vi "RMET.vi"(2 "Run uninterrupted?":bool, 3 "Device Category IN:":string(combo)="Mini" caption="Device Category:", 5 "Sensor Serial No. IN:":string caption="Sensor Serial No.:", 6 "DB Serial No. IN:":string caption="DB Serial No.:") -> (0 "Done!":bool)   [LabVIEW 2019]
doc: "Performs IV measurements according to ATLAS ITk Quality Control Specifications."
uses:
  general_VIs/globals/QC_MeasurementSetup.vi
  general_VIs/globals/QC_RunInformation.vi
  InstrControl/InstrumentSetup.vi
  InstrControl/Switching/Switching.lvclass
  InstrControl/SupplyControl/SupplyControl.lvclass
  InstrControl/ArduinoControl/ArduinoControl.lvclass
  <vilib>/Analysis/NI_AALBase.lvlib
  InstrControl/InstrControl.lvclass
panel:
  out "Measurement Configuration Tab":enum32{"R_MET Setup", "R_MET Scan"}(tab)
  in  "Set voltage limit?":bool
  in  "Voltage Limit [mV]":dbl=1000.0 min=0.0001 format="%.3f"
  in  "Measurement Configurations":bool
  in  "Initial volts [uA] IN":dbl caption="Initial volts [V]"
  in  "Final volts [uA] IN":dbl=-700.0 caption="Final volts [V]"
  in  "step [uA] IN":dbl=10.0 caption="step [V]" format="%.1f"
  in  "step interval [s] IN":i32=10 caption="step interval [s]"
  in  "Continue":bool
  in  "Quit":bool
  out "RH":dbl[](array[numeric]) caption="RH [%]" format="%#.2f"
  out "Temp.":dbl[](array[numeric]) caption="Temp. [°C]" format="%#.2f"
  out "Resistance":dbl[](array[numeric]) caption="Resistance [Ohms]"
  out "Current":dbl[](array[numeric]) caption="Current [uA]"
  out "step interval [s]":i32=10
  out "step [V]":dbl=10.0 format="%.1f"
  out "Final volts [V]":dbl=-700.0 format="%.1f"
  out "Initial volts [V]":dbl format="%.1f"
  out "Igraph":cluster{dbl[], dbl[]}(graph)
  in  "Scales":T1(ring)
  in  "Iscale":enum16{"Ohms", "kiloOhms", "MegaOhms"}(ring)
  out "positive ramp?":bool
  out "DUT Description/Hardware Tab":enum32{"R_MET Setup", "R_MET Scan"}(tab)
  in  "Structure Name IN:":string caption="Structure Name:"
  in  "Switching":string(combo)="LXIPXI Switching"
  in  "Hardware Configurations":bool
  in  "User:":string(combo)="Xavi"
  in  "IV Supply":string(combo)="Keithley 2410"
  in  "Temperature":enum16{"Read Arduino", "Enter manually"}(ring)
  in  "Manufacturer:":string(combo)="Hamamatsu"
  out "Structure Name":string caption="Structure Name:"
  in  "abort":bool
  out "Device Category:":string
  out "DB Serial No.:":string
  out "Current Volts:":dbl format="%.2f"
  in  "quit (no save)":bool
  in  "Quit & Save":bool
  out "Bias On/Off:":bool
  out "STATUS 1":string
  out "Initiated:":string
  out "Sensor No.:":string
  out "No of steps":u32
  out "Current reading No.":u32
  out "Last reading at:":string
  # "University of\nCambridge"
  # "Strip Sensor QC: Metal Resistance"
  # "Vertical Scale:"
  # "Measurement Configuration"
  # "Scan parameters:"
  # "Last 5 readings:"
  # "n-4"
  # "n-3"
  # "n-2"
  # "n-1"
  # "n"
  # "DUT Description"
  # "Hardware"
  # "DUT & Test Description:"
  # "Current status:"
  # "Rdg No:"
  # "out of"
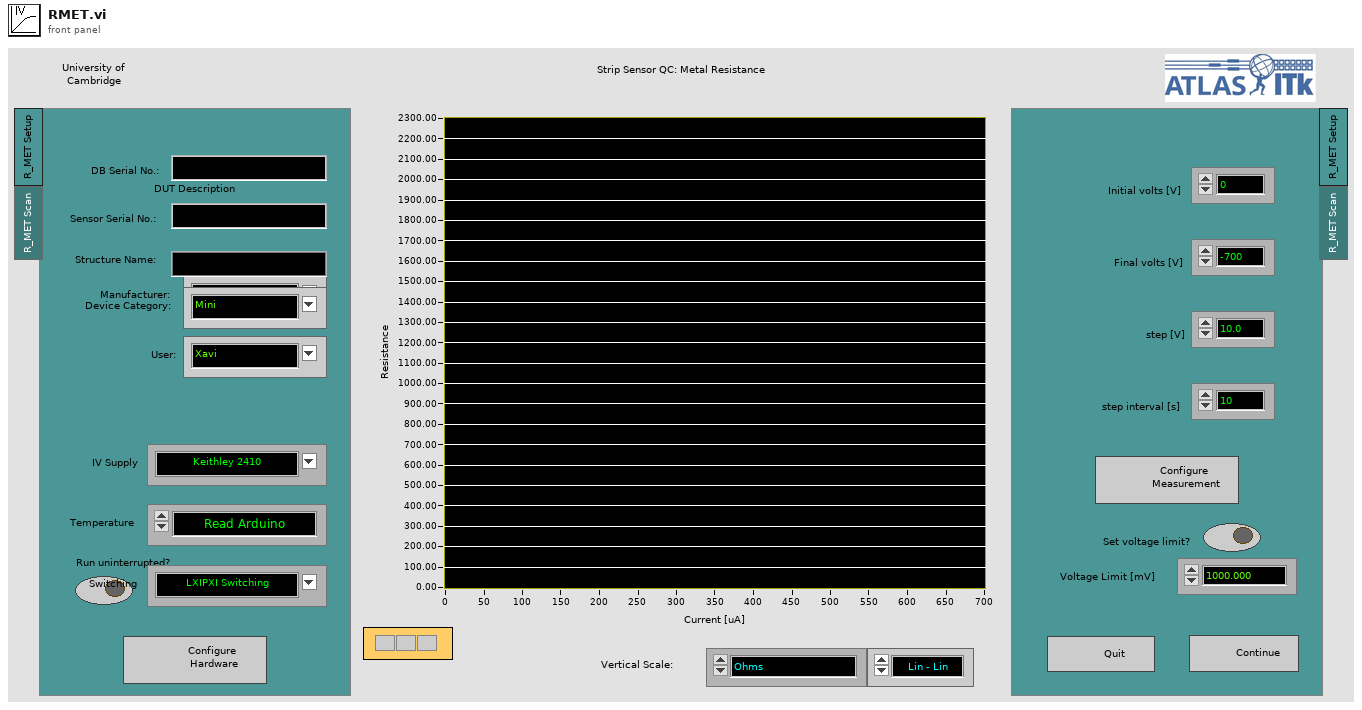
[diagram p1: front panel]
types:
  T1 = enum16{"Lin - Lin", "Log - Lin", "Lin - Log", "Log - log"}
  T2 = enum16{"Supply", "LCR", "Multimeter", "Switching"}
  T3 = enum16{"Reset", "Read Array", "Read Element", "Write Element", "Write Array", "Add Element", "Add Array"}
  T4 = enum16{"Reset", "Ground", "Striptest Bias", "Striptest SMU", "Striptest LCR", "IV", "CV", "Interstrip Cap", "Interstrip Res"}
  T5 = enum16{"Reset", "Ground", "Striptest Bias", "Striptest SMU", "Striptest LCR", "IV", "CV", "Interstrip Cap", "Interstrip Res", "PTP", "Implant Resistance", "Metal Resistance", "Coupling Capacitance"}
  T6 = cluster{"Supply":refnum<class "SupplyControl.lvclass">, "Initial Current [uA]":dbl, "Final Current [uA]":dbl, "Step Size [uA]":dbl, "Step Interval [s]":i32, "Number Of Steps":u32, "Ramp down steps [uA]":dbl, "Ramp down Interval [s]":i32, "Set Current Limit?":bool, "Voltage Limit [mV]":dbl, "Temperature Readout":enum16{"Read Arduino", "Enter manually"}, "Arduino":refnum<class "ArduinoControl.lvclass">, "Supply Name":string, "Switching":refnum<class "Switching.lvclass">, "Matrix used?":bool, "Matrix X Channels":cluster{"Bias Supply / SMU LO":i32, "Bias Supply / SMU HI":i32, "CV Box LO":i32, "CV Box HI":i32, "CV Box LO IN":i32, "CV Box HI IN":i32, "Volt meter LO":i32, "Volt meter HI":i32, "Mux1 C1":i32, "Mux1 C2":i32, "Mux2 C1":i32, "Mux2 C2":i32}, "Structure Name":string}
  T7 = cluster{"Sensor Serial No.:":string, "Wafer Serial No.:":string, "Batch:":string, "Manufacturer:":string, "Device Category:":string, "Database Serial No.:":string, "Date Initiated:":string, "Time Initiated:":string, "Test":string, "Instruments used:":string, "Probeplan used:":string, "End of Run comment:":string, "User:":string}
  T8 = cluster{"Institute":string, "Manufacturers":string[], "Devices":string[], "Serialnumbers Lookup DB":string, "Data directory":string, "Backup & screenshot directory":string, "List of known users":string[], "Measurement switch not used":bool, "Measurement Switch":string, "DUT Switch":string}
  T9 = cluster{"Supply":refnum<class "SupplyControl.lvclass">, "Initial Voltage [V]":dbl, "Final Voltage [V]":dbl, "Step Size [V]":dbl, "Step Interval [s]":i32, "Number Of Steps":u32, "Ramp down steps [V]":dbl, "Ramp down Interval [s]":i32, "Set Current Limit?":bool, "Current Limit [µA]":dbl, "Temperature Readout":enum16{"Read Arduino", "Enter manually"}, "Arduino":refnum<class "ArduinoControl.lvclass">, "Supply Name":string, "Switching":refnum<class "Switching.lvclass">, "Matrix used?":bool, "Matrix X Channels":cluster{"Bias Supply / SMU LO":i32, "Bias Supply / SMU HI":i32, "CV Box LO":i32, "CV Box HI":i32, "CV Box LO IN":i32, "CV Box HI IN":i32, "Volt meter LO":i32, "Volt meter HI":i32, "Mux1 C1":i32, "Mux1 C2":i32, "Mux2 C1":i32, "Mux2 C2":i32}, "Structure Name":string}
  T10 = cluster{"Voltage Limit":sgl, "R_Metal_KE2410":refnum<class "R_Metal_KE2410.lvclass">}
  T11 = cluster{"VISA address":refnum<visa-resource-name>, "T sensor":enum16{"SHT", "DS"}, "Arduino":refnum<class "ArduinoControl.lvclass">}
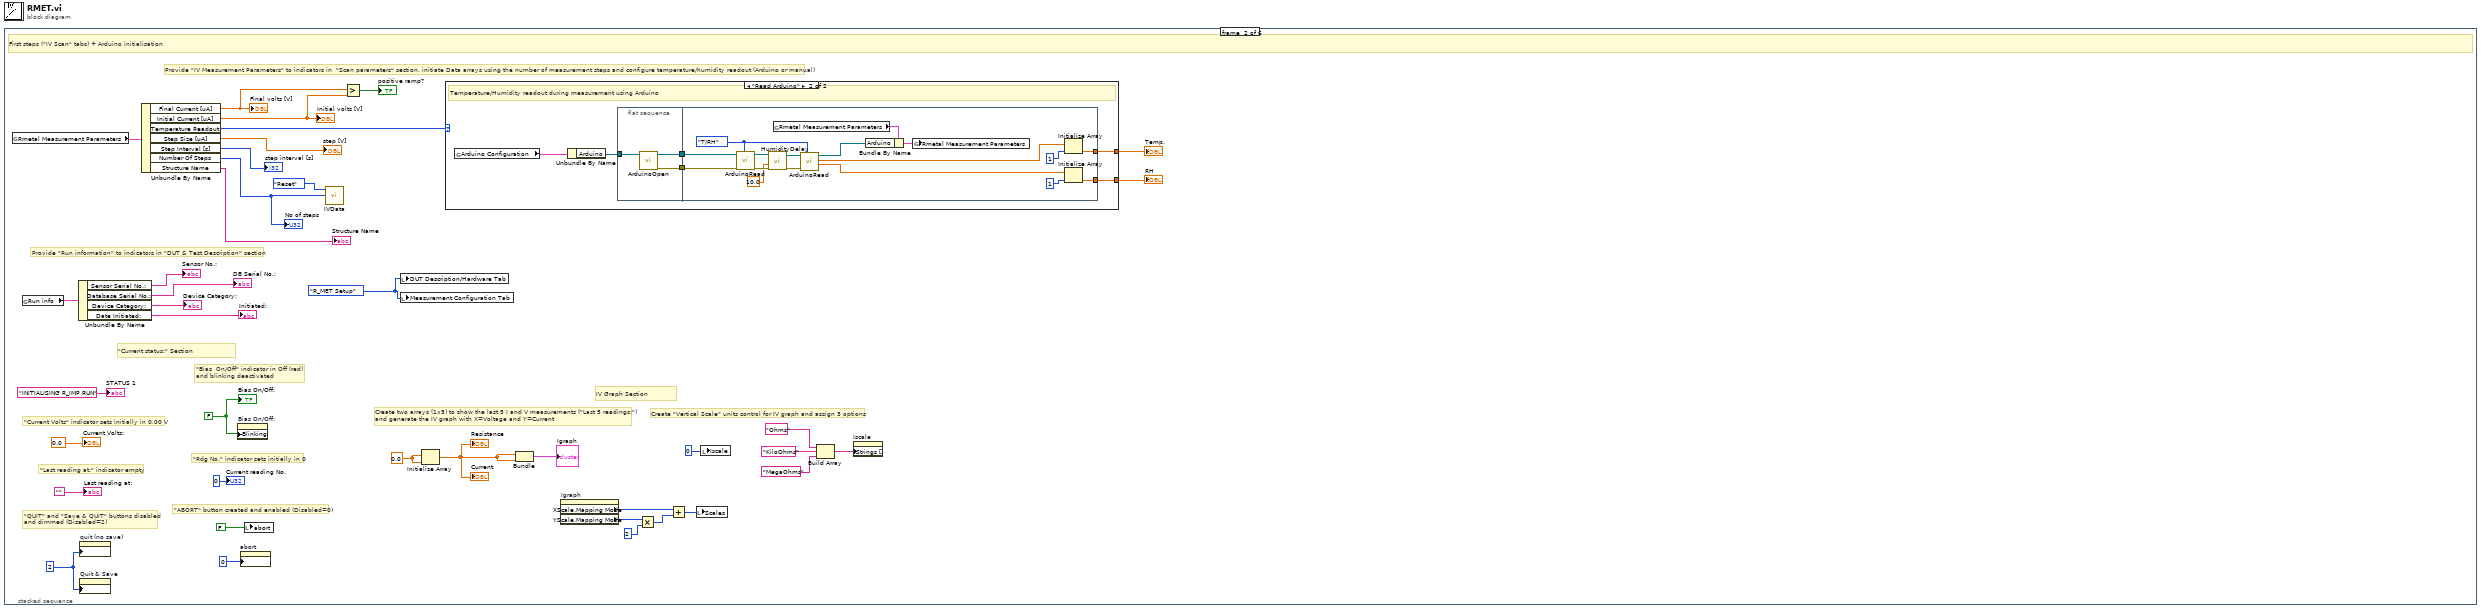
[diagram p0: block diagram]
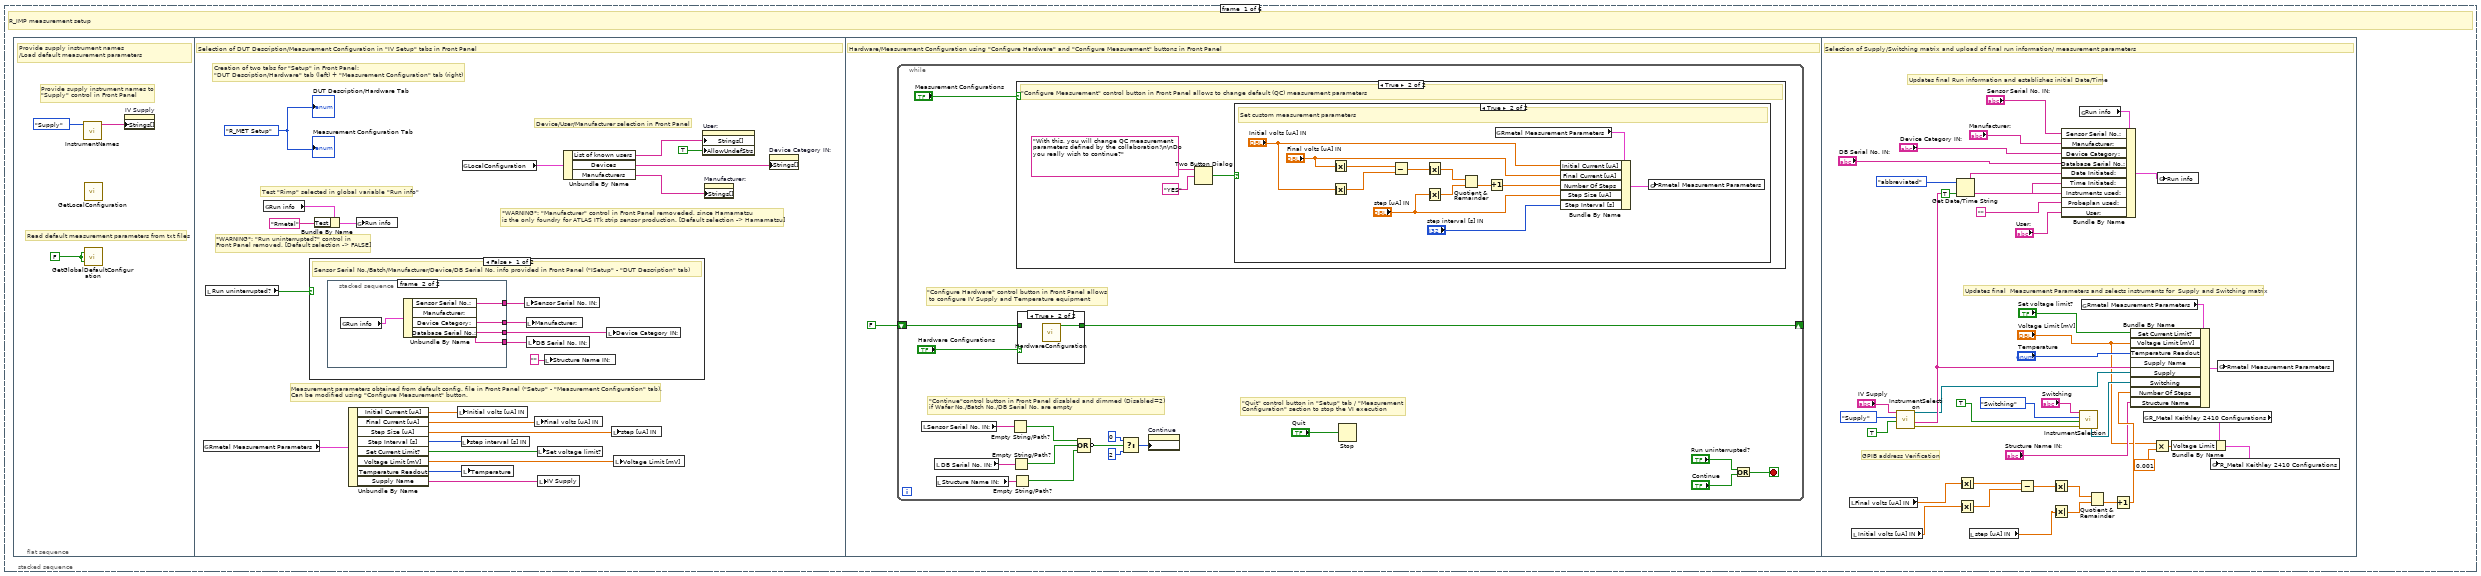
[diagram p2: hidden frame]
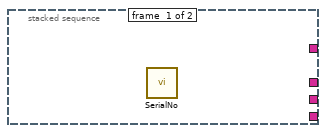
[diagram p3: hidden frame]
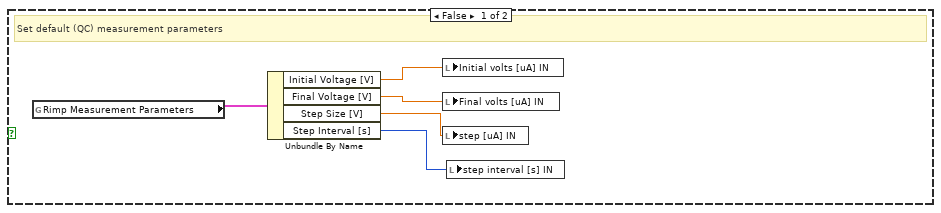
[diagram p6: hidden frame]
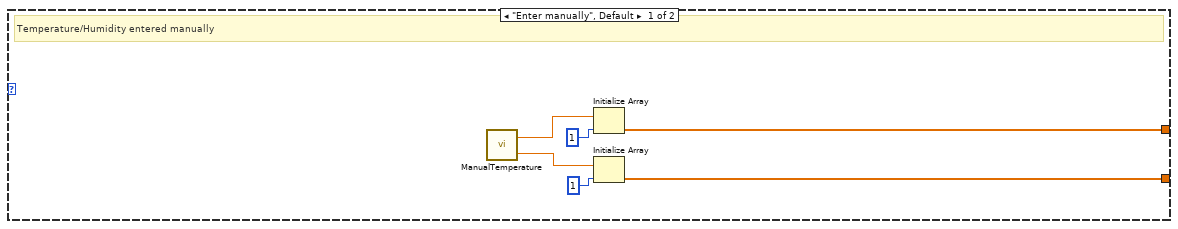
[diagram p8: hidden frame]
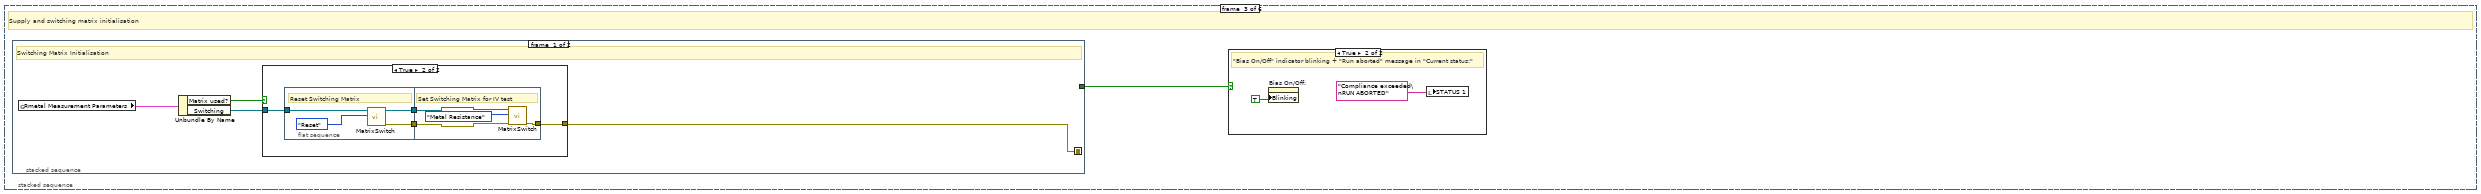
[diagram p9: hidden frame]
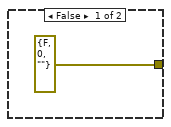
[diagram p10: hidden frame]
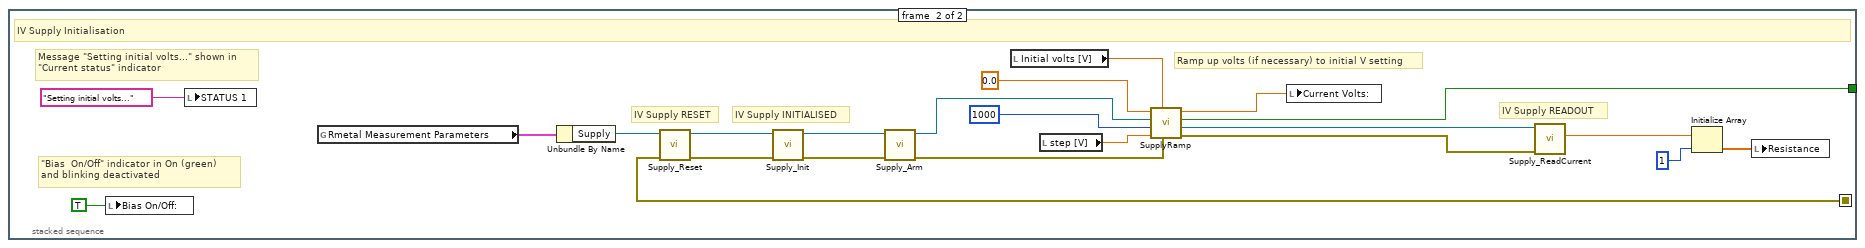
[diagram p11: hidden frame]
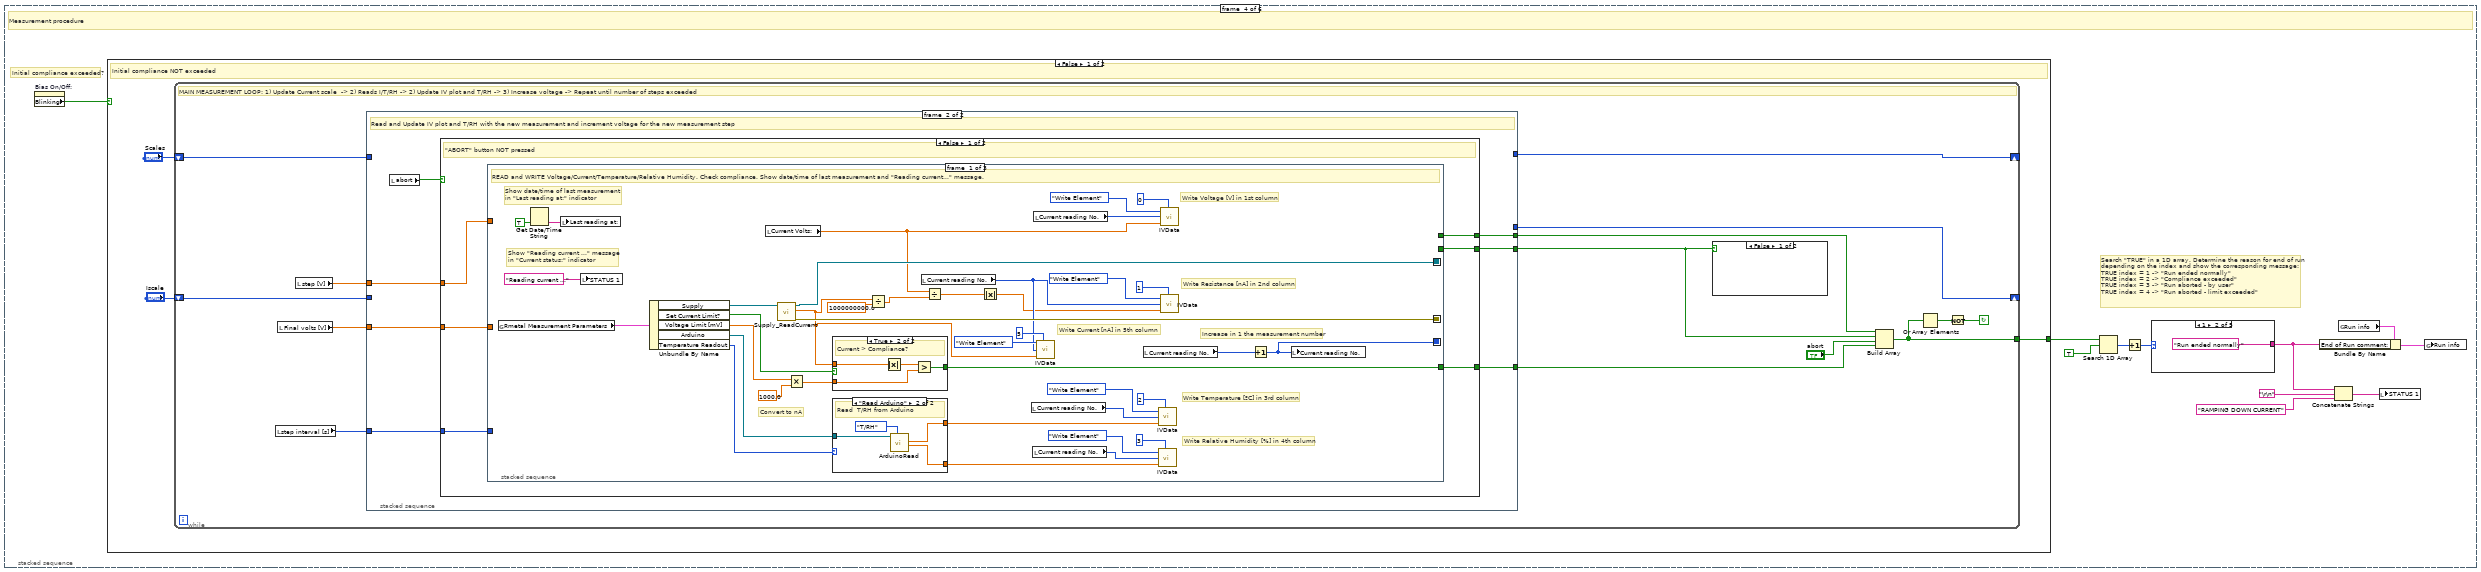
[diagram p13: hidden frame]
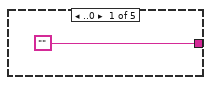
[diagram p14: hidden frame]
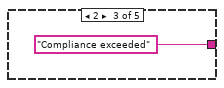
[diagram p15: hidden frame]
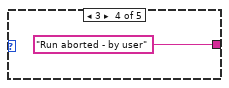
[diagram p16: hidden frame]
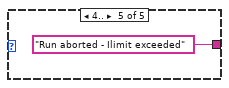
[diagram p17: hidden frame]
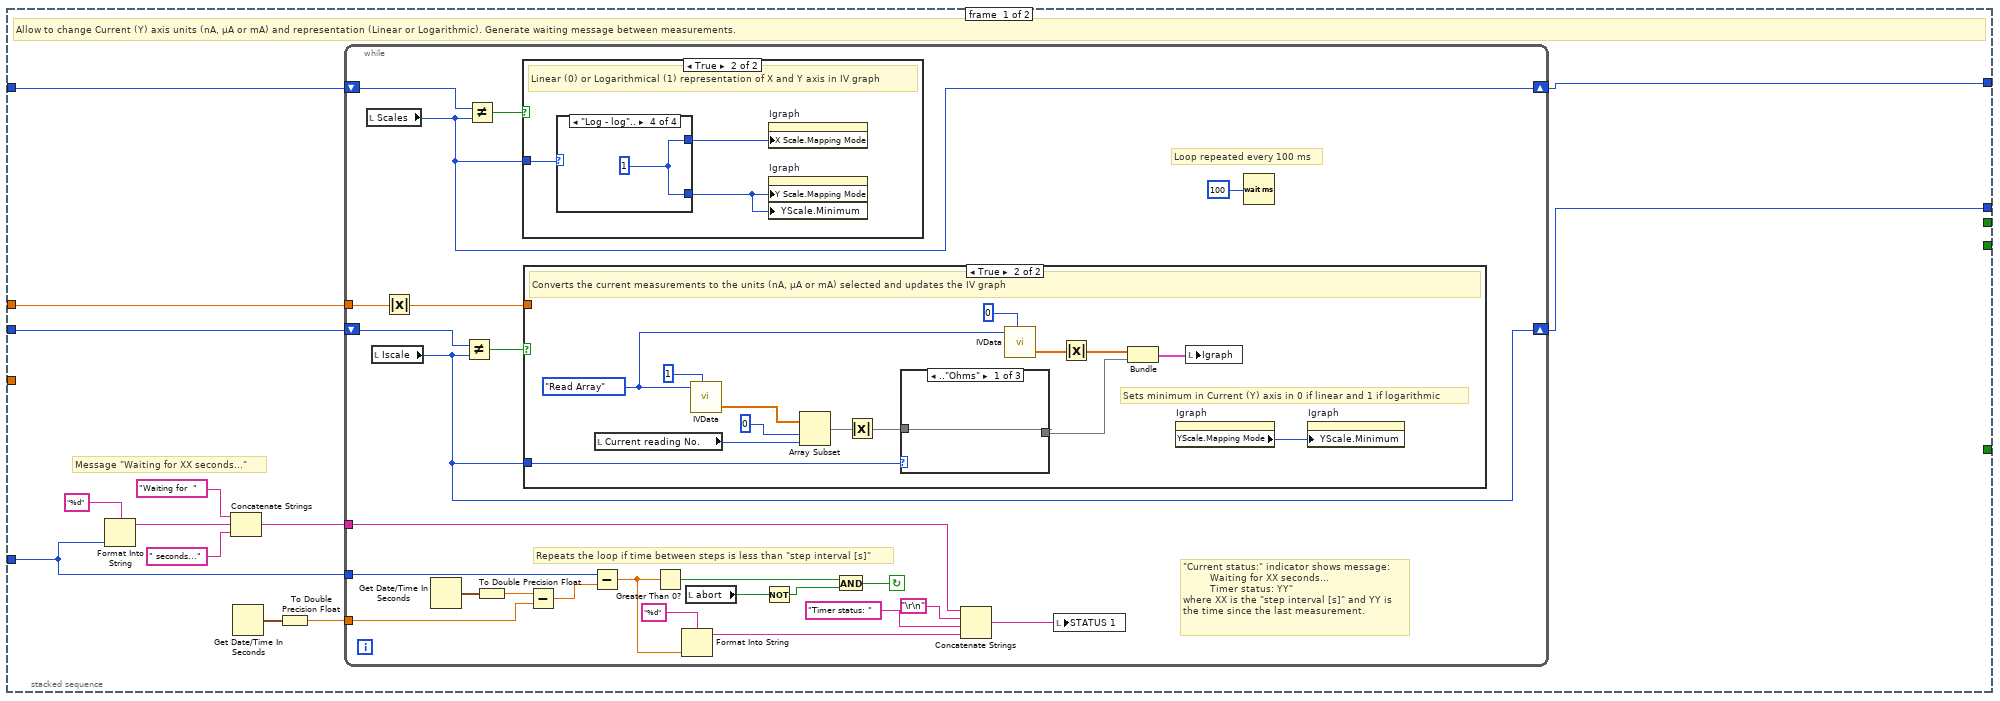
[diagram p18: hidden frame]
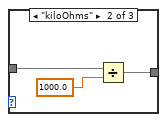
[diagram p20: hidden frame]
diagram:
  n1 = stacked-sequence {
    frame #0 {
      # "R_IMP measurement setup"
      n2 = flat-sequence {
        frame #0 {
          w3 = FALSE
          # "Read default measurement parameters from txt files"
          # "Provide supply instrument names to \n\"Supply\" control in Front Panel"
          # "Provide supply instrument names\n/Load default measurement parameters"
          n3 = call "InstrumentNames.vi"("Instrument type"=T2."Supply") -> ("Instrument names"=w1:string[])  [unwired: 9 in, 1 out]
          n4 = call "GetLocalConfiguration.vi"() -> ()  [unwired: 3 in, 1 out]
          n5 = call "GetGlobalDefaultConfiguration.vi"("DO NOT override instruments"=w3, "Read defaults?"=w3) -> ()  [unwired: 1 in, 1 out]
          n6 = property on="IV Supply" class="CmbBox"("Strings[]"=w1) -> ()  [unwired: 2 in, 2 out]
        }
        frame #1 {
          w4 = enum32{"R_MET Setup", "R_MET Scan"}."R_MET Setup" ("DUT Description/Hardware Tab")
          # "Device/User/Manufacturer selection in Front Panel"
          # "*WARNING*: \"Manufacturer\" control in Front Panel removeded, since Hamamatsu \nis the only foundry for ATLAS ITk strip sensor production. [Default selection -> Hamamatsu]"
          # "Measurement parameters obtained from default config. file in Front Panel (\"Setup\" - \"Measurement Configuration\" tab).\nCan be modified using \"Configure Measurement\" button."
          # "Test \"Rimp\" selected in global variable \"Run info\""
          # "Creation of two tabs for \"Setup\" in Front Panel:\n\"DUT Description/Hardware\" tab (left) + \"Measurement Configuration\" tab (right)"
          # "*WARNING*: \"Run uninterrupted?\" control in \nFront Panel removed. [Default selection -> FALSE]"
          # "Selection of DUT Description/Measurement Configuration in \"IV Setup\" tabs in Front Panel"
          n7 = global read "QC_MeasurementSetup.vi" "Rmetal Measurement Parameters"() -> (w20:T6)
          n8 = local read "Run uninterrupted?"() -> (w14:bool)
          n9 = global read "QC_RunInformation.vi" "Run info"() -> (w13:T7)
          n10 = case shown="False" w14 {
            frame False {
              # "Sensor Serial No./Batch/Manufacturer/Device/DB Serial No. info provided in Front Panel (\"ISetup\" - \"DUT Description\" tab)"
              n11 = stacked-sequence {
                tunnel: [_ w32] -> w26
                tunnel: [_ w31] -> w25
                tunnel: [_ w30] -> w27
                tunnel: [_ w28] -> w24
                frame #0 {
                  n12 = call "SerialNo.vi"() -> ()  [unwired: 5 in, 1 out]
                }
                frame #1 {
                  n13 = global read "QC_RunInformation.vi" "Run info"() -> (w29:T7)
                  n14 = Unbundle By Name(w29) -> ("Sensor Serial No.:"=w32:string, "Manufacturer:"=w31:string, "Device Category:"=w30:string, "Database Serial No.:"=w28:string)
                }
              }
              n15 = local write "Sensor Serial No. IN:"(w26) -> ()
              n16 = local write "Manufacturer:"(w25) -> ()
              n17 = local write "DB Serial No. IN:"(w24) -> ()
              n18 = local write "Structure Name IN:"("" ("Structure Name IN:")) -> ()
              n19 = local write "Device Category IN:"(w27) -> ()
            }
            frame True {
            }
          }
          n20 = Bundle By Name(cluster=w13, "Test"="Rmetal") -> (w12:T7)
          n21 = Unbundle By Name(w20) -> ("Initial Current [uA]"=w10:dbl, "Final Current [uA]"=w9:dbl, "Step Size [uA]"=w8:dbl, "Step Interval [s]"=w11:i32, "Set Current Limit?"=w19:bool, "Voltage Limit [mV]"=w18:dbl, "Temperature Readout"=w22:enum16{"Read Arduino", "Enter manually"}, "Supply Name"=w21:string)
          n22 = global write "QC_RunInformation.vi" "Run info"(w12) -> ()
          n23 = local write "Initial volts [uA] IN"(w10) -> ()
          n24 = local write "step interval [s] IN"(w11) -> ()
          n25 = local write "Temperature"(w22) -> ()
          n26 = global read "QC_RunInformation.vi" "LocalConfiguration"() -> (w17:T8)
          n27 = local write "Final volts [uA] IN"(w9) -> ()
          n28 = local write "Set voltage limit?"(w19) -> ()
          n29 = local write "IV Supply"(w21) -> ()
          n30 = Unbundle By Name(w17) -> ("List of known users"=w16:string[], "Devices"=w7:string[], "Manufacturers"=w6:string[])
          n31 = local write "step [uA] IN"(w8) -> ()
          n32 = local write "Voltage Limit [mV]"(w18) -> ()
          n33 = property on="User:" class="CmbBox"("Strings[]"=w16, "AllowUndefStrs"=TRUE) -> ()  [unwired: 2 in, 2 out]
          n34 = property on="Manufacturer:" class="CmbBox"("Strings[]"=w6) -> ()  [unwired: 2 in, 2 out]
          n35 = property on="Device Category IN:" class="CmbBox"("Strings[]"=w7) -> ()  [unwired: 2 in, 2 out]
          "DUT Description/Hardware Tab" <- w4
          "Measurement Configuration Tab" <- w4
        }
        frame #2 {
          # "Hardware/Measurement Configuration using \"Configure Hardware\" and \"Configure Measurement\" buttons in Front Panel"
          n36 = while {
            shift-right: [w43] -> _
            shift-left: FALSE -> [w42]
            stop <- w39 stop-if-true
            # "\"Continue\"control button in Front Panel disabled and dimmed (Disabled=2) \nif Wafer No./Batch No./DB Serial No. are empty"
            # "\"Configure Hardware\" control button in Front Panel allows\n to configure IV Supply and Temperature equipment"
            # "\"Quit\" control button in \"Setup\" tab / \"Measurement \nConfiguration\" section to stop the VI execution"
            n37 = local read "Sensor Serial No. IN:"() -> (w50:string)
            n38 = local read "DB Serial No. IN:"() -> (w37:string)
            n39 = local read "Structure Name IN:"() -> (w35:string)
            n40 = Empty String/Path?(string/path=w50) -> (empty?=w49:bool)
            n41 = Empty String/Path?(string/path=w37) -> (empty?=w36:bool)
            n42 = Empty String/Path?(string/path=w35) -> (empty?=w34:bool)
            n43 = case shown="True" "Measurement Configurations" {
              frame False {
              }
              frame True {
                # "\"Configure Measurement\" control button in Front Panel allows to change default (QC) measurement parameters"
                n44 = Two Button Dialog(message="With this, you will change QC measurement parameters defined by the collaboration!\n\nDo you really wish to continue?", 2:"YES") -> (T button?=w52:bool)  [unwired: 1 in]
                n45 = case shown="True" w52 {
                  frame False {
                    # "Set default (QC) measurement parameters"
                    n46 = global read "QC_MeasurementSetup.vi" "Rimp Measurement Parameters"() -> (w59:T9)
                    n47 = Unbundle By Name(w59) -> ("Initial Voltage [V]"=w57:dbl, "Final Voltage [V]"=w58:dbl, "Step Size [V]"=w56:dbl, "Step Interval [s]"=w55:i32)
                    n48 = local write "Initial volts [uA] IN"(w57) -> ()
                    n49 = local write "Final volts [uA] IN"(w58) -> ()
                    n50 = local write "step [uA] IN"(w56) -> ()
                    n51 = local write "step interval [s] IN"(w55) -> ()
                  }
                  frame True {
                    # "Set custom measurement parameters"
                    n52 = Absolute Value(x="Final volts [uA] IN") -> (abs(x)=w70:dbl)
                    n53 = Absolute Value(x="Initial volts [uA] IN") -> (abs(x)=w69:dbl)
                    n54 = Subtract(x=w70, y=w69) -> (x-y=w64:dbl)
                    n55 = Absolute Value(x=w64) -> (abs(x)=w66:dbl)
                    n56 = Absolute Value(x="step [uA] IN") -> (abs(x)=w65:dbl)
                    n57 = Quotient & Remainder(x=w66, y=w65) -> (floor(x/y)=w63:dbl)  [unwired: 1 out]
                    n58 = Increment(x=w63) -> (x+1=w62:dbl)
                    n59 = global read "QC_MeasurementSetup.vi" "Rmetal Measurement Parameters"() -> (w72:T6)
                    n60 = Bundle By Name(cluster=w72, "Initial Current [uA]"="Initial volts [uA] IN", "Final Current [uA]"="Final volts [uA] IN", "Number Of Steps"=w62, "Step Size [uA]"="step [uA] IN", "Step Interval [s]"="step interval [s] IN") -> (w71:T6)
                    n61 = global write "QC_MeasurementSetup.vi" "Rmetal Measurement Parameters"(w71) -> ()
                  }
                }
              }
            }
            n62 = case shown="True" "Hardware Configurations" {
              tunnel: [w73 w74] -> w43
              tunnel: w42 -> [w73 _]
              frame False {
              }
              frame True {
                n63 = call "HardwareConfiguration.vi"() -> ("configured?"=w74:bool)  [unwired: 11 in]
              }
            }
            n64 = Compound Arithmetic op=OR(w49, w36, w34) -> (invert w48:bool)
            n65 = Select(t=0, s=w48, f=2) -> (s? t:f=w45:i32)
            n66 = property on="Continue" class="Bool"("DisabledEnum"=w45) -> ()  [unwired: 2 in, 2 out]
            n67 = Stop(stop? (T)="Quit") -> ()
            n68 = Or(x="Run uninterrupted?", y="Continue") -> (x .or. y?=w39:bool)
          }
        }
        frame #3 {
          # "GPIB address Verification"
          # "Updates final  Measurement Parameters and selects instruments for  Supply and Switching matrix"
          # "Updates final Run information and establishes initial Date/Time"
          # "Selection of Supply/Switching matrix and upload of final run information/ measurement parameters"
          n69 = local read "Final volts [uA] IN"() -> (w82:dbl)
          n70 = local read "Initial volts [uA] IN"() -> (w83:dbl)
          n71 = call "InstrumentSelection.vi"("Verify GPIB address"=TRUE, "Instrument type"=T2."Supply", "Instrument name IN"="IV Supply") -> ("error out"=w100:errorcluster, "Instrument name OUT"=w103:string, "Supply"=w102:refnum<class "SupplyControl.lvclass">)  [unwired: 3 in, 3 out]
          n72 = Get Date/Time String(date format (0)=enum16{"short", "long", "abbreviated"}."abbreviated", want seconds? (F)=TRUE) -> (date string=w94:string, time string=w93:string)  [unwired: 1 in]
          n73 = Absolute Value(x=w82) -> (abs(x)=w90:dbl)
          n74 = Absolute Value(x=w83) -> (abs(x)=w89:dbl)
          n75 = local read "step [uA] IN"() -> (w84:dbl)
          n76 = Subtract(x=w90, y=w89) -> (x-y=w86:dbl)
          n77 = Absolute Value(x=w86) -> (abs(x)=w88:dbl)
          n78 = Absolute Value(x=w84) -> (abs(x)=w87:dbl)
          n79 = global read "QC_RunInformation.vi" "Run info"() -> (w111:T7)
          n80 = Bundle By Name(cluster=w111, "Sensor Serial No.:"="Sensor Serial No. IN:", "Manufacturer:"="Manufacturer:", "Device Category:"="Device Category IN:", "Database Serial No.:"="DB Serial No. IN:", "Date Initiated:"=w94, "Time Initiated:"=w93, "Instruments used:"=w103, "Probeplan used:"="", "User:"="User:") -> (w110:T7)
          n81 = call "InstrumentSelection.vi"("error in (no error)"=w100, "Verify GPIB address"=TRUE, "Instrument type"=T2."Switching", "Instrument name IN"="Switching") -> ("Switching"=w99:refnum<class "Switching.lvclass">)  [unwired: 2 in, 5 out]
          n82 = global read "QC_MeasurementSetup.vi" "Rmetal Measurement Parameters"() -> (w115:T6)
          n83 = Quotient & Remainder(x=w88, y=w87) -> (floor(x/y)=w85:dbl)  [unwired: 1 out]
          n84 = Increment(x=w85) -> (x+1=w81:dbl)
          n85 = Bundle By Name(cluster=w115, "Set Current Limit?"="Set voltage limit?", "Voltage Limit [mV]"="Voltage Limit [mV]", "Temperature Readout"="Temperature", "Supply Name"=w103, "Supply"=w102, "Switching"=w99, "Number Of Steps"=w81, "Structure Name"="Structure Name IN:") -> (w116:T6)
          n86 = global read "InstrumentSetup.vi" "R_Metal Keithley 2410 Configurations"() -> (w79:T10)
          n87 = Multiply(x="Voltage Limit [mV]", y=0.001) -> (x*y=w76:dbl)
          n88 = global write "QC_RunInformation.vi" "Run info"(w110) -> ()
          n89 = Bundle By Name(cluster=w79, "Voltage Limit"=w76) -> (w78:T10)
          n90 = global write "InstrumentSetup.vi" "R_Metal Keithley 2410 Configurations"(w78) -> ()
          n91 = global write "QC_MeasurementSetup.vi" "Rmetal Measurement Parameters"(w116) -> ()
        }
      }
    }
    frame #1 {
      w117 = enum32{"R_MET Setup", "R_MET Scan"}."R_MET Setup" ("DUT Description/Hardware Tab")
      w139 = 2
      w145 = 0.0
      w138 = FALSE ("Visible")
      # "IV Graph Section"
      # "\"Current status:\" Section"
      # "Create two arrays (1x5) to show the last 5 I and V measurements (\"Last 5 readings:\") \nand generate the IV graph with X=Voltage and Y=Current"
      # "\"Bias  On/Off\" indicator in Off (red)\nand blinking deactivated"
      # "\"Rdg No.\" indicator sets initially in 0"
      # "\"ABORT\" button created and enabled (Disabled=0)"
      # "\"Current Volts\" indicator sets initially in 0.00 V"
      # "\"Last reading at:\" indicator empty"
      # "\"QUIT\" and \"Save & QUIT\" buttons disabled\nand dimmed (Disabled=2)"
      # "Create \"Vertical Scale\" units control for IV graph and assign 3 options"
      # "Provide \"Run information\" to indicators in \"DUT & Test Description\" section"
      # "Provide \"IV Measurement Parameters\" to indicators in  \"Scan parameters\" section, initiate Data arrays using the number of measurement steps and configure temperature/humidity readout (Arduino or manual)"
      # "First steps (\"IV Scan\" tabs) + Arduino initialisation"
      n92 = global read "QC_MeasurementSetup.vi" "Rmetal Measurement Parameters"() -> (w129:T6)
      n93 = global read "QC_RunInformation.vi" "Run info"() -> (w154:T7)
      n94 = Unbundle By Name(w154) -> ("Sensor Serial No.:"=→"Sensor No.:":string, "Database Serial No.:"=→"DB Serial No.:":string, "Device Category:"=→"Device Category:":string, "Date Initiated:"=→"Initiated:":string)
      n95 = property on="quit (no save)" class="Bool"("DisabledEnum"=w139) -> ()  [unwired: 2 in, 2 out]
      n96 = property on="Quit & Save" class="Bool"("DisabledEnum"=w139) -> ()  [unwired: 2 in, 2 out]
      n97 = Unbundle By Name(w129) -> ("Final Current [uA]"=w121:dbl, "Initial Current [uA]"=w122:dbl, "Temperature Readout"=w123:enum16{"Read Arduino", "Enter manually"}, "Step Size [uA]"=→"step [V]":dbl, "Step Interval [s]"=→"step interval [s]":i32, "Number Of Steps"=w119:u32, "Structure Name"=→"Structure Name":string)
      "No of steps" <- w119
      "Initial volts [V]" <- w122
      "Final volts [V]" <- w121
      n98 = property on="Bias On/Off:" class="Bool (strict)"("Blinking"=w138) -> ()  [unwired: 2 in, 2 out]
      n99 = property on="abort" class="Bool (strict)"("DisabledEnum"=0) -> ()  [unwired: 2 in, 2 out]
      n100 = local write "abort"(FALSE) -> ()
      n101 = call "IVData.vi"("Action"=T3."Reset", "Array Size / Index"=w119) -> ()  [unwired: 3 in, 2 out]
      n102 = Greater?(x=w121, y=w122) -> (0:→"positive ramp?":bool)
      n103 = local write "DUT Description/Hardware Tab"(w117) -> ()
      n104 = local write "Measurement Configuration Tab"(w117) -> ()
      n105 = Initialize Array(w145, w145) -> (w125:dbl[])
      "Current" <- w125
      "Resistance" <- w125
      n106 = case shown="\"Read Arduino\"" w123 {
        tunnel: [w160 w167] -> w142
        tunnel: [w157 w166] -> w130
        frame "Enter manually", Default {
          # "Temperature/Humidity entered manually"
          n107 = call "ManualTemperature.vi"() -> ("Humidity [%] out"=w156:dbl, "Temperature [°C] out"=w161:dbl)
          n108 = Initialize Array(w161, 1) -> (w160:dbl[])
          n109 = Initialize Array(w156, 1) -> (w157:dbl[])
        }
        frame "Read Arduino" {
          # "Temperature/Humidity readout during measurement using Arduino"
          n110 = global read "InstrumentSetup.vi" "Arduino Configuration"() -> (w163:T11)
          n111 = Unbundle By Name(w163) -> ("Arduino"=w162:refnum<class "ArduinoControl.lvclass">)
          n112 = flat-sequence {
            tunnel: [w168] -> w165
            tunnel: [w170] -> w164
            tunnel: w162 -> [w169]
            tunnel: [w187] -> w167
            tunnel: [w184] -> w166
            tunnel: w165 -> [w178]
            tunnel: w164 -> [w177]
            frame #0 {
              n113 = call "ArduinoOpen.vi"("ArduinoControl in"=w169) -> ("error out"=w170:errorcluster, "ArduinoControl out"=w168:refnum<class "ArduinoControl.lvclass">)  [unwired: 9 in]
            }
            frame #1 {
              w176 = enum16{"T/RH", "Interlock", "Edgesense"}."T/RH" ("Arduino function")
              n114 = call "ArduinoRead.vi"("Arduino function"=w176, "error in (no error)"=w177, "ArduinoControl in"=w178) -> ("error out"=w172:errorcluster, "ArduinoControl out"=w173:refnum<class "ArduinoControl.lvclass">)  [unwired: 3 in, 4 out]
              n115 = call "HumidityDelay.vi"("error in (no error)"=w172, "Start Humidity"=10.0, "ArduinoControl in"=w173) -> ("error out"=w175:errorcluster, "ArduinoControl out"=w174:refnum<class "ArduinoControl.lvclass">)  [unwired: 7 in]
              n116 = global read "QC_MeasurementSetup.vi" "Rmetal Measurement Parameters"() -> (w180:T6)
              n117 = call "ArduinoRead.vi"("Arduino function"=w176, "error in (no error)"=w175, "ArduinoControl in"=w174) -> ("rel. Humidity [%]"=w182:dbl, "Temperature [°C]"=w183:dbl, "ArduinoControl out"=w181:refnum<class "ArduinoControl.lvclass">)  [unwired: 3 in, 3 out]
              n118 = Bundle By Name(cluster=w180, "Arduino"=w181) -> (w179:T6)
              n119 = global write "QC_MeasurementSetup.vi" "Rmetal Measurement Parameters"(w179) -> ()
              n120 = Initialize Array(w183, 1) -> (w187:dbl[])
              n121 = Initialize Array(w182, 1) -> (w184:dbl[])
            }
          }
        }
      }
      "Temp." <- w142
      "RH" <- w130
      n122 = Bundle(w125, w125) -> (→"Igraph":cluster{dbl[], dbl[]})  [unwired: 1 in]
      n123 = property on="Igraph" class="XYGraph (strict)"() -> ("XScale.Mapping Mode"=w133:u8, "YScale.Mapping Mode"=w132:u8)  [unwired: 2 in, 2 out]
      n124 = Multiply(x=w132, y=2) -> (x*y=w135:i32)
      n125 = Add(x=w133, y=w135) -> (x+y=w131:i32)
      n126 = local write "Scales"(w131) -> ()
      n127 = local write "Iscale"(u16 0 ("Scale")) -> ()
      n128 = Build Array("Ohms", "KiloOhms", "MegaOhms") -> (w151:string[])
      n129 = property on="Iscale" class="Enum (strict)"("Strings []"=w151) -> ()  [unwired: 2 in, 2 out]
      "STATUS 1" <- "INITIALISING R_IMP RUN"
      "Bias On/Off:" <- w138
      "Last reading at:" <- ""
      "Current reading No." <- u32 0 ("Current reading No.")
      "Current Volts:" <- 0.0 ("Current Volts:")
    }
    frame #2 {
      # "Supply and switching matrix initialisation"
      n130 = stacked-sequence {
        seq-local: [w190 _] -> [_ w206]
        tunnel: [_ w207] -> w188
        frame #0 {
          # "Switching Matrix Initialisation"
          n131 = global read "QC_MeasurementSetup.vi" "Rmetal Measurement Parameters"() -> (w189:T6)
          n132 = Unbundle By Name(w189) -> ("Matrix used?"=w192:bool, "Switching"=w191:refnum<class "Switching.lvclass">)
          n133 = case shown="True" w192 {
            tunnel: w191 -> [_ w194]
            tunnel: [errorcluster {"status"=FALSE, "code"=0, "source"=""} ("error constant") w195] -> w190
            frame False {
            }
            frame True {
              n134 = flat-sequence {
                tunnel: [w201] -> w197
                tunnel: [w200] -> w196
                tunnel: w194 -> [w199]
                tunnel: w197 -> [w205]
                tunnel: w196 -> [w204]
                tunnel: [w203] -> w195
                frame #0 {
                  # "Reset Switching Matrix"
                  n135 = call-dynamic "MatrixSwitch.vi"("Action"=T4."Reset", "Switching in"=w199) -> ("error out"=w201:errorcluster, "Switching out"=w200:refnum<class "Switching.lvclass">)  [unwired: 7 in, 1 out]
                }
                frame #1 {
                  # "Set Switching Matrix for IV test"
                  n136 = call-dynamic "MatrixSwitch.vi"("error in (no error)"=w205, "Action"=T5."Metal Resistance", "Switching in"=w204) -> ("error out"=w203:errorcluster)  [unwired: 6 in, 2 out]
                }
              }
            }
          }
        }
        frame #1 {
          # "IV Supply READOUT"
          # "IV Supply INITIALISED"
          # "IV Supply RESET"
          # "Message \"Setting initial volts...\" shown in \n\"Current status\" indicator"
          # "\"Bias  On/Off\" indicator in On (green)\nand blinking deactivated"
          # "Ramp up volts (if necessary) to initial V setting"
          # "IV Supply Initialisation"
          n137 = local write "Bias On/Off:"(TRUE ("Compliance?")) -> ()
          n138 = local write "STATUS 1"("Setting initial volts..." ("STATUS 1")) -> ()
          n139 = global read "QC_MeasurementSetup.vi" "Rmetal Measurement Parameters"() -> (w223:T6)
          n140 = Unbundle By Name(w223) -> ("Supply"=w220:refnum<class "SupplyControl.lvclass">)
          n141 = call-dynamic "Supply_Reset.vi"("error in (no error)"=w206, "SupplyControl in"=w220) -> ("error out"=w225:errorcluster, "SupplyControl out"=w227:refnum<class "SupplyControl.lvclass">)  [unwired: 8 in]
          n142 = call-dynamic "Supply_Init.vi"("error in (no error)"=w225, "SupplyControl in"=w227) -> ("error out"=w224:errorcluster, "SupplyControl out"=w226:refnum<class "SupplyControl.lvclass">)  [unwired: 8 in]
          n143 = call-dynamic "Supply_Arm.vi"("error in (no error)"=w224, "SupplyControl in"=w226) -> ("error out"=w213:errorcluster, "SupplyControl out"=w214:refnum<class "SupplyControl.lvclass">)  [unwired: 8 in]
          n144 = local read "Initial volts [V]"() -> (w215:dbl)
          n145 = local read "step [V]"() -> (w216:dbl)
          n146 = call "SupplyRamp.vi"("error in"=w213, "Requested Voltage"=w215, "Step Size"=w216, "Step Delay"=1000, "Supply IN"=w214, "Starting Voltage"=0.0) -> ("error out"=w208:errorcluster, "Supply OUT"=w209:refnum<class "SupplyControl.lvclass">, "Compliance exceeded"=w207:bool, "Current Voltage"=w219:dbl)  [unwired: 2 in]
          n147 = local write "Current Volts:"(w219) -> ()
          n148 = call-dynamic "Supply_ReadCurrent.vi"("error in (no error)"=w208, "SupplyControl in"=w209) -> ("Current in nA"=w211:dbl)  [unwired: 7 in, 2 out]
          n149 = Initialize Array(w211, 1) -> (w210:dbl[])
          n150 = local write "Resistance"(w210) -> ()
        }
      }
      n151 = case shown="True" w188 {
        frame False {
        }
        frame True {
          # "\"Bias On/Off\" indicator blinking + \"Run aborted\" message in \"Current status:\""
          n152 = property on="Bias On/Off:" class="Bool (strict)"("Blinking"=TRUE) -> ()  [unwired: 2 in, 2 out]
          n153 = local write "STATUS 1"("Compliance exceeded\nRUN ABORTED") -> ()
        }
      }
    }
    frame #3 {
      # "Search \"TRUE\" in a 1D array. Determine the reason for end of run \ndepending on the index and show the corresponding message:\nTRUE index = 1 -> \"Run ended normally\"\nTRUE index = 2 -> \"Compliance exceeded\"\nTRUE index = 3 -> \"Run aborted - by user\"\nTRUE index = 4 -> \"Run aborted - limit exceeded\""
      # "Initial compliance exceeded?"
      # "Measurement procedure"
      n154 = property on="Bias On/Off:" class="Bool (strict)"() -> ("Blinking"=w240:bool)  [unwired: 2 in, 2 out]
      n155 = case shown="False" w240 {
        tunnel: [w248 w494] -> w239
        frame False {
          # "Initial compliance NOT exceeded"
          n156 = while {
            shift-left: "Iscale" -> [w258]
            shift-right: [w257] -> _
            shift-left: "Scales" -> [w259]
            shift-right: [w260] -> _
            tunnel: [w256] -> w248
            stop <- w261 continue-if-true
            # "MAIN MEASUREMENT LOOP: 1) Update Current scale  -> 2) Reads I/T/RH -> 2) Update IV plot and T/RH -> 3) Increase voltage -> Repeat until number of steps exceeded"
            n157 = local read "step interval [s]"() -> (w253:i32)
            n158 = local read "Final volts [V]"() -> (w254:dbl)
            n159 = local read "step [V]"() -> (w255:dbl)
            n160 = stacked-sequence {
              tunnel: [w275 _] -> w260
              tunnel: w255 -> [w272 w337]
              tunnel: [_ w336] -> w251
              tunnel: w254 -> [_ w335]
              tunnel: w253 -> [w263 w334]
              tunnel: [_ w333] -> w252
              tunnel: w259 -> [w274 _]
              tunnel: w258 -> [w273 _]
              tunnel: [w271 _] -> w257
              tunnel: [_ w331] -> w249
              frame #0 {
                # "Message \"Waiting for XX seconds...\""
                # "Allow to change Current (Y) axis units (nA, µA or mA) and representation (Linear or Logarithmic). Generate waiting message between measurements."
                n161 = Format Into String(format string="%d", w263) -> (resulting string=w268:string)  [unwired: 2 in, 1 out]
                n162 = Concatenate Strings("Waiting for  ", w268, " seconds...") -> (w264:string)
                n163 = Get Date/Time In Seconds() -> (seconds since 1Jan1904=w265:timestamp)
                n164 = To Double Precision Float(number=w265) -> (double precision float=w266:dbl)
                n165 = while {
                  tunnel: w272 -> [w284]
                  shift-left: w273 -> [w288]
                  shift-right: [w281] -> w271
                  shift-left: w274 -> [w289]
                  shift-right: [w290] -> w275
                  tunnel: w264 -> [w282]
                  tunnel: w263 -> [w294]
                  tunnel: w266 -> [w295]
                  stop <- w296 continue-if-true
                  # "\"Current status:\" indicator shows message:\n         Waiting for XX seconds...\n         Timer status: YY\"\nwhere XX is the \"step interval [s]\" and YY is\nthe time since the last measurement."
                  # "Repeats the loop if time between steps is less than \"step interval [s]\""
                  # "Loop repeated every 100 ms"
                  n166 = local read "Scales"() -> (w290:T1)
                  n167 = local read "Iscale"() -> (w281:enum16{"Ohms", "kiloOhms", "MegaOhms"})
                  n168 = Absolute Value(x=w284) -> (abs(x)=w283:dbl)
                  n169 = Get Date/Time In Seconds() -> (seconds since 1Jan1904=w280:timestamp)
                  n170 = Not Equal?(x=w288, y=w281) -> (x != y?=w279:bool)
                  n171 = Not Equal?(x=w289, y=w290) -> (x != y?=w291:bool)
                  n172 = To Double Precision Float(number=w280) -> (double precision float=w300:dbl)
                  n173 = case shown="True" w291 {
                    tunnel: w290 -> [_ w324]
                    frame False {
                    }
                    frame True {
                      # "Linear (0) or Logarithmical (1) representation of X and Y axis in IV graph"
                      n174 = case shown="\"Log - log\".." w324 {
                        tunnel: [w325 1 0 w330] -> w323
                        tunnel: [w325 0 1 w330] -> w322
                        frame .."Lin - Lin" {
                          w325 = 0
                        }
                        frame "Log - Lin" {
                        }
                        frame "Lin - Log" {
                        }
                        frame "Log - log".. {
                          w330 = 1
                        }
                      }
                      n175 = property on="Igraph" class="XYGraph (strict)"("X Scale.Mapping Mode"=w323) -> ()  [unwired: 2 in, 2 out]
                      n176 = property on="Igraph" class="XYGraph (strict)"("Y Scale.Mapping Mode"=w322, "YScale.Minimum"=w322) -> ()  [unwired: 2 in, 2 out]
                    }
                  }
                  n177 = case shown="True" w279 {
                    tunnel: w283 -> [_ _]
                    tunnel: w281 -> [_ w309]
                    frame False {
                    }
                    frame True {
                      w303 = T3."Read Array" ("Action")
                      # "Sets minimum in Current (Y) axis in 0 if linear and 1 if logarithmic"
                      # "Converts the current measurements to the units (nA, µA or mA) selected and updates the IV graph"
                      n178 = local read "Current reading No."() -> (w311:u32)
                      n179 = call "IVData.vi"("Action"=w303, "Array No."=u32 1 ("Action")) -> ("Array OUT"=w312:dbl[])  [unwired: 3 in, 1 out]
                      n180 = Array Subset(array=w312, index=0, length=w311) -> (w308:dbl[])
                      n181 = Absolute Value(x=w308) -> (abs(x)=w307:dbl[])
                      n182 = case shown="..\"Ohms\"" w309 {
                        tunnel: [w315 w316 w320] -> w314
                        tunnel: w307 -> [w315 w318 w321]
                        frame .."Ohms" {
                        }
                        frame "kiloOhms" {
                          n183 = Divide(x=w318, y=1000.0) -> (x/y=w316:dbl[])
                        }
                        frame "MegaOhms".. {
                          n184 = Divide(x=w321, y=1000000.0) -> (x/y=w320:dbl[])
                        }
                      }
                      n185 = call "IVData.vi"("Action"=w303, "Array No."=u32 0 ("Action")) -> ("Array OUT"=w302:dbl[])  [unwired: 3 in, 1 out]
                      n186 = Absolute Value(x=w302) -> (abs(x)=w301:dbl[])
                      n187 = Bundle(w301, w314) -> (w310:cluster{dbl[], dbl[]})  [unwired: 1 in]
                      n188 = property on="Igraph" class="XYGraph (strict)"() -> ("YScale.Mapping Mode"=w305:u8)  [unwired: 2 in, 2 out]
                      n189 = local write "Igraph"(w310) -> ()
                      n190 = property on="Igraph" class="XYGraph (strict)"("YScale.Minimum"=w305) -> ()  [unwired: 2 in, 2 out]
                    }
                  }
                  n191 = Subtract(x=w300, y=w295) -> (x-y=w277:dbl)
                  n192 = Subtract(x=w294, y=w277) -> (x-y=w276:dbl)
                  n193 = Greater Than 0?(x=w276) -> (x > 0?=w278:bool)
                  n194 = Format Into String(format string="%d", w276) -> (resulting string=w298:string)  [unwired: 2 in, 1 out]
                  n195 = local read "abort"() -> (w293:bool)
                  n196 = Not(x=w293) -> (.not. x?=w299:bool)
                  n197 = And(x=w278, y=w299) -> (x .and. y?=w296:bool)
                  n198 = Concatenate Strings(w282, "\r\n", "Timer status: ", w298) -> (w292:string)
                  n199 = local write "STATUS 1"(w292) -> ()
                  n200 = Wait (ms)(milliseconds to wait=u32 100) -> ()  [unwired: 1 out]
                }
              }
              frame #1 {
                # "Read and Update IV plot and T/RH with the new measurement and increment voltage for the new measurement step"
                n201 = local read "abort"() -> (w332:bool)
                n202 = case shown="False" w332 {
                  tunnel: [w343 w491] -> w333
                  tunnel: w334 -> [w342 _]
                  tunnel: w335 -> [w341 _]
                  tunnel: [w339 w491] -> w336
                  tunnel: w337 -> [w340 _]
                  tunnel: [w338 w491] -> w331
                  frame False {
                    # "\"ABORT\" button NOT pressed"
                    n203 = stacked-sequence {
                      seq-local: [w354 _ _] -> [_ w401 _]
                      seq-local: [w371 _ _] -> [_ _ w460]
                      seq-local: [w370 _ _] -> [_ _ w461]
                      tunnel: w340 -> [_ _ w466]
                      tunnel: w341 -> [_ _ w458]
                      tunnel: [_ _ w464] -> w343
                      tunnel: [_ _ w463] -> w339
                      tunnel: w342 -> [_ _ _]
                      tunnel: [w377 _ _] -> w338
                      frame #0 {
                        # "Write Current [nA] in 5th column"
                        # "Write Relative Humidity [%] in 4th column"
                        # "Write Temperature [ºC] in 3rd column"
                        # "Write Resistance [nA] in 2nd column"
                        # "Write Voltage [V] in 1st column"
                        # "Increase in 1 the measurement number"
                        # "Convert to nA"
                        # "Show \"Reading current ...\" message \nin \"Current status:\" indicator"
                        # "Show date/time of last measurement \nin \"Last reading at:\" indicator"
                        # "READ and WRITE Voltage/Current/Temperature/Relative Humidity. Check compliance. Show date/time of last measurement and \"Reading current...\" message."
                        n204 = global read "QC_MeasurementSetup.vi" "Rmetal Measurement Parameters"() -> (w369:T6)
                        n205 = Get Date/Time String(want seconds? (F)=TRUE) -> (time string=w374:string)  [unwired: 2 in, 1 out]
                        n206 = local write "Last reading at:"(w374) -> ()
                        n207 = local write "STATUS 1"("Reading current ..." ("status")) -> ()
                        n208 = Unbundle By Name(w369) -> ("Supply"=w364:refnum<class "SupplyControl.lvclass">, "Set Current Limit?"=w368:bool, "Voltage Limit [mV]"=w366:dbl, "Arduino"=w362:refnum<class "ArduinoControl.lvclass">, "Temperature Readout"=w363:enum16{"Read Arduino", "Enter manually"})
                        n209 = local read "Current Volts:"() -> (w352:dbl)
                        n210 = call-dynamic "Supply_ReadCurrent.vi"("SupplyControl in"=w364) -> ("error out"=w370:errorcluster, "Current in nA"=w345:dbl, "SupplyControl out"=w371:refnum<class "SupplyControl.lvclass">)  [unwired: 8 in]
                        n211 = Multiply(x=w366, y=1000.0) -> (x*y=w365:dbl)
                        n212 = case shown="True" w368 {
                          tunnel: w345 -> [_ w396]
                          tunnel: w365 -> [_ w394]
                          tunnel: [FALSE w393] -> w377
                          frame False {
                            # "Measurement without compliance"
                          }
                          frame True {
                            # "Current > Compliance?"
                            n213 = Absolute Value(x=w396) -> (abs(x)=w395:dbl)
                            n214 = Greater?(x=w395, y=w394) -> (0:w393:bool)
                          }
                        }
                        n215 = case shown="\"Read Arduino\"" w363 {
                          tunnel: [w385 w391] -> w375
                          tunnel: [w382 w390] -> w372
                          tunnel: w362 -> [_ w389]
                          frame "Enter manually", Default {
                            # "Read T/RH entered manually"
                            n216 = local read "Temp."() -> (w387:dbl[])
                            n217 = local read "RH"() -> (w383:dbl[])
                            n218 = Index Array(array=w387, index=0) -> (element=w385:dbl)
                            n219 = Index Array(array=w383, index=0) -> (element=w382:dbl)
                          }
                          frame "Read Arduino" {
                            # "Read  T/RH from Arduino"
                            n220 = call "ArduinoRead.vi"("Arduino function"=enum16{"T/RH", "Interlock", "Edgesense"}."T/RH", "ArduinoControl in"=w389) -> ("rel. Humidity [%]"=w390:dbl, "Temperature [°C]"=w391:dbl)  [unwired: 4 in, 4 out]
                          }
                        }
                        n221 = Divide(x=w345, y=1000000000.0) -> (x/y=w350:dbl)
                        n222 = local read "Current reading No."() -> (w346:u32)
                        n223 = Divide(x=w352, y=w350) -> (x/y=w349:dbl)
                        n224 = Absolute Value(x=w349) -> (abs(x)=w344:dbl)
                        n225 = local read "Current reading No."() -> (w359:u32)
                        n226 = local read "Current reading No."() -> (w353:u32)
                        n227 = local read "Current reading No."() -> (w360:u32)
                        n228 = call "IVData.vi"("Action"=T3."Write Element", "Array No."=u32 5, "Array Size / Index"=w346, "Data IN"=w345) -> ()  [unwired: 1 in, 2 out]
                        n229 = local read "Current reading No."() -> (w355:u32)
                        n230 = call "IVData.vi"("Action"=T3."Write Element", "Array No."=u32 2, "Array Size / Index"=w359, "Data IN"=w375) -> ()  [unwired: 1 in, 2 out]
                        n231 = call "IVData.vi"("Action"=T3."Write Element", "Array No."=u32 3, "Array Size / Index"=w353, "Data IN"=w372) -> ()  [unwired: 1 in, 2 out]
                        n232 = call "IVData.vi"("Action"=T3."Write Element", "Array No."=0, "Array Size / Index"=w360, "Data IN"=w352) -> ()  [unwired: 1 in, 2 out]
                        n233 = call "IVData.vi"("Action"=T3."Write Element", "Array No."=u32 1, "Array Size / Index"=w346, "Data IN"=w344) -> ()  [unwired: 1 in, 2 out]
                        n234 = Increment(x=w355) -> (x+1=w354:u32)
                        n235 = local write "Current reading No."(w354) -> ()
                      }
                      frame #1 {
                        w399 = T3."Read Array" ("Action")
                        w411 = u32 5 ("y")
                        # "Update Current/Voltage plots"
                        # "Set minimum in Current (Y) axis in 0 if linear and 1 if logarithmic"
                        # "Update IV plot and show Temperature/Relative Humidity and last 5 readings of Current/Voltage"
                        n236 = call "IVData.vi"("Action"=w399, "Array No."=0) -> ("Array OUT"=w398:dbl[])  [unwired: 3 in, 1 out]
                        n237 = call "IVData.vi"("Action"=w399, "Array No."=1) -> ("Array OUT"=w413:dbl[])  [unwired: 3 in, 1 out]
                        n238 = Absolute Value(x=w398) -> (abs(x)=w397:dbl[])
                        n239 = Array Subset(array=w413, index=0, length=w401) -> (w406:dbl[])
                        n240 = Greater?(x=w401, y=w411) -> (0:w410:bool)
                        n241 = local read "Iscale"() -> (w412:enum16{"Ohms", "kiloOhms", "MegaOhms"})
                        n242 = Absolute Value(x=w406) -> (abs(x)=w405:dbl[])
                        n243 = case shown="False" w410 {
                          tunnel: w401 -> [w417 w420]
                          tunnel: w411 -> [_ w419]
                          tunnel: [w417 w419] -> w409
                          tunnel: [0 w418] -> w407
                          frame False {
                          }
                          frame True {
                            n244 = Subtract(x=w420, y=w419) -> (x-y=w418:u32)
                          }
                        }
                        n245 = property on="Igraph" class="XYGraph (strict)"() -> ("YScale.Mapping Mode"=w402:u8)  [unwired: 2 in, 2 out]
                        n246 = case shown="..\"Ohms\"" w412 {
                          tunnel: [w445 w446 w449] -> w415
                          tunnel: w405 -> [w445 w448 w451]
                          frame .."Ohms" {
                          }
                          frame "kiloOhms" {
                            n247 = Divide(x=w448, y=1000.0) -> (x/y=w446:dbl[])
                          }
                          frame "MegaOhms".. {
                            n248 = Divide(x=w451, y=1000000.0) -> (x/y=w449:dbl[])
                          }
                        }
                        n249 = property on="Igraph" class="XYGraph (strict)"("YScale.Minimum"=w402) -> ()  [unwired: 2 in, 2 out]
                        n250 = for {
                          N: 4 -> [_]
                          tunnel: w409 -> [w425]
                          tunnel: w407 -> [w424]
                          tunnel: w401 -> [w421]
                          i -> [w426]
                          # "Update \"Last 5 readings:\" IV indicator and T/RH indicators"
                          n251 = call "IVData.vi"("Action"=T3."Read Array", "Array No."=w426) -> ("Array OUT"=w423:dbl[])  [unwired: 3 in, 1 out]
                          n252 = case shown="3.." w426 {
                            tunnel: w425 -> [w429 w433 _ _]
                            tunnel: w424 -> [w430 w434 _ _]
                            tunnel: w423 -> [w428 w432 w438 w443]
                            tunnel: w421 -> [_ _ w436 w441]
                            frame ..0 {
                              # "Read Voltage from 1st column"
                              n253 = Array Subset(array=w428, index=w430, length=w429) -> (w427:dbl[])
                              n254 = local write "Current"(w427) -> ()
                            }
                            frame 1 {
                              # "Read Current from 2nd column"
                              n255 = Array Subset(array=w432, index=w434, length=w433) -> (w431:dbl[])
                              n256 = local write "Resistance"(w431) -> ()
                            }
                            frame 2 {
                              # "Read Temperature from 3rd column"
                              n257 = Decrement(x=w436) -> (x-1=w435:u32)
                              n258 = Array Subset(array=w438, index=w435, length=1) -> (w437:dbl[])
                              n259 = local write "Temp."(w437) -> ()
                            }
                            frame 3.. {
                              # "Read Relative Humidity from 4th column"
                              n260 = Decrement(x=w441) -> (x-1=w440:u32)
                              n261 = Array Subset(array=w443, index=w440, length=1) -> (w442:dbl[])
                              n262 = local write "RH"(w442) -> ()
                            }
                          }
                        }
                        n263 = Bundle(w397, w415) -> (w403:cluster{dbl[], dbl[]})  [unwired: 1 in]
                        n264 = local write "Igraph"(w403) -> ()
                      }
                      frame #2 {
                        # "Increase volts and check for end of ramp"
                        # "Increase voltage and check compliance"
                        n265 = local read "Current Volts:"() -> (w453:dbl)
                        n266 = local read "Current Volts:"() -> (w452:dbl)
                        n267 = local read "positive ramp?"() -> (w462:bool)
                        n268 = Quotient & Remainder(x=w452, y=w458) -> (x-y*floor(x/y)=w459:dbl, floor(x/y)=w457:dbl)
                        n269 = case shown="False" w462 {
                          tunnel: w458 -> [w469 w473]
                          tunnel: w466 -> [w470 w476]
                          tunnel: [w468 w475] -> w454
                          tunnel: [w467 w472] -> w465
                          tunnel: w453 -> [w471 w474]
                          frame False {
                            n270 = Subtract(x=w471, y=w470) -> (x-y=w467:dbl)
                            n271 = Greater Or Equal?(x=w467, y=w469) -> (x >= y?=w468:bool)
                          }
                          frame True {
                            n272 = Add(x=w474, y=w476) -> (x+y=w472:dbl)
                            n273 = Less Or Equal?(x=w472, y=w473) -> (x <= y?=w475:bool)
                          }
                        }
                        n274 = Not Equal To 0?(x=w459) -> (x != 0?=w455:bool)
                        n275 = Equal To 0?(x=w457) -> (x = 0?=w456:bool)
                        n276 = Or(x=w455, y=w456) -> ()  [unwired: 1 out]
                        n277 = case shown="True" w454 {
                          tunnel: w465 -> [_ w488]
                          tunnel: [TRUE FALSE] -> w464
                          tunnel: [FALSE w479] -> w463
                          tunnel: w452 -> [_ w486]
                          tunnel: w461 -> [_ w485]
                          tunnel: w460 -> [_ w484]
                          frame False {
                          }
                          frame True {
                            # "Message \"Incrementing volts.\""
                            # "Increase  voltage, check compliance and check PTP supply errors"
                            n278 = local read "step [V]"() -> (w482:dbl)
                            n279 = call "SupplyRamp.vi"("error in"=w485, "Requested Voltage"=w488, "Step Size"=w482, "Step Delay"=100, "Supply IN"=w484, "Starting Voltage"=w486) -> ("error out"=w480:errorcluster, "Compliance exceeded"=w479:bool, "Current Voltage"=w483:dbl)  [unwired: 2 in, 1 out]
                            n280 = local write "STATUS 1"("Incrementing volts.") -> ()
                            n281 = case shown="No Error" w480 {
                              tunnel: w483 -> [w490 _]
                              frame No Error {
                                n282 = local write "Current Volts:"(w490) -> ()
                              }
                              frame Error {
                              }
                            }
                            n283 = property on="Bias On/Off:" class="Bool (strict)"("Blinking"=w479) -> ()  [unwired: 2 in, 2 out]
                          }
                        }
                      }
                    }
                  }
                  frame True {
                    w491 = FALSE
                    # "\"ABORT\" button pressed"
                  }
                }
              }
            }
            n284 = case shown="False" w251 {
              frame False {
              }
              frame True {
                n285 = property on="Bias On/Off:" class="Bool (strict)"("Blinking"=TRUE) -> ()  [unwired: 2 in, 2 out]
              }
            }
            n286 = Build Array(w252, w251, "abort", w249) -> (w256:bool[])
            n287 = Or Array Elements(Boolean array=w256) -> (logical OR=w262:bool)
            n288 = Not(x=w262) -> (.not. x?=w261:bool)
          }
        }
        frame True {
          w493 = FALSE
          # "Flag compliance as reason for end of run"
          # "Compliance exceeded when first voltage applied"
          n289 = local write "STATUS 1"("Run aborted - compliance exceeded.") -> ()
          n290 = Build Array(w493, TRUE, w493, w493) -> (w494:bool[])
        }
      }
      n291 = Search 1D Array(1D array=w239, element=TRUE) -> (index of element=w237:i32)  [unwired: 1 in]
      n292 = Increment(x=w237) -> (x+1=w236:i32)
      n293 = case shown="1" w236 {
        tunnel: ["" "Run ended normally" "Compliance exceeded" "Run aborted - by user" "Run aborted - Ilimit exceeded"] -> w231
        frame ..0 {
        }
        frame 1 {
        }
        frame 2 {
        }
        frame 3 {
        }
        frame 4.. {
        }
      }
      n294 = Concatenate Strings(w231, "\r\n", "RAMPING DOWN CURRENT") -> (w234:string)
      n295 = global read "QC_RunInformation.vi" "Run info"() -> (w235:T7)
      n296 = Bundle By Name(cluster=w235, "End of Run comment:"=w231) -> (w230:T7)
      n297 = local write "STATUS 1"(w234) -> ()
      n298 = global write "QC_RunInformation.vi" "Run info"(w230) -> ()
    }
    frame #4 {
      # "Ramp down, switch off supply, ask to save data and save jpg of the Front Panel"
      n299 = stacked-sequence {
        frame #0 {
          # "Switch IV supply to STANDBY"
          # "s -> ms"
          # "Ramp down voltage and switch IV supply to standby"
          n300 = global read "QC_MeasurementSetup.vi" "Rmetal Measurement Parameters"() -> (w505:T6)
          n301 = Unbundle By Name(w505) -> ("Supply"=w504:refnum<class "SupplyControl.lvclass">, "Ramp down Interval [s]"=w497:i32, "Ramp down steps [uA]"=w498:dbl, "Switching"=w499:refnum<class "Switching.lvclass">, "Matrix used?"=w500:bool)
          n302 = local read "Current Volts:"() -> (w510:dbl)
          n303 = Multiply(x=w497, y=1000) -> (x*y=w507:i32)
          n304 = call "SupplyRamp.vi"("Requested Voltage"=0.0, "Step Size"=w498, "Step Delay"=w507, "Supply IN"=w504, "Starting Voltage"=w510) -> ("error out"=w503:errorcluster, "Supply OUT"=w502:refnum<class "SupplyControl.lvclass">, "Current Voltage"=w508:dbl)  [unwired: 3 in, 1 out]
          n305 = local write "Current Volts:"(w508) -> ()
          n306 = call-dynamic "Supply_Stby.vi"("error in (no error)"=w503, "SupplyControl in"=w502) -> ("error out"=w501:errorcluster)  [unwired: 8 in, 1 out]
          n307 = case shown="True" w500 {
            tunnel: w499 -> [_ w515]
            tunnel: w501 -> [_ w514]
            frame False {
            }
            frame True {
              # "CLOSE Switching Matrix"
              # "RESET Switching  Matrix"
              n308 = call-dynamic "MatrixSwitch.vi"("error in (no error)"=w514, "Action"=T4."Reset", "Switching in"=w515) -> ("error out"=w511:errorcluster, "Switching out"=w512:refnum<class "Switching.lvclass">)  [unwired: 6 in, 1 out]
              n309 = call-dynamic "Close.vi"("error in (no error)"=w511, "Switching in"=w512) -> ()  [unwired: 8 in, 2 out]
            }
          }
        }
        frame #1 {
          w520 = 0
          # "\"Current Volts\" indicator back to 0.00 V"
          # "\"Bias  On/Off\" indicator in Off (red)"
          # "\"ABORT\" button disanabled \nand dimmed (Disabled=2)"
          # "\"QUIT\" and \"Save & QUIT\" buttons \nenabled (Disabled=0)"
          # "Reset \"Current Volts\" and \"Bias On/Off\" indicators, \"ABORT\" button disabled and \"QUIT\"/\"Save & QUIT\" buttons enabled"
          n310 = property on="Quit & Save" class="Bool"("DisabledEnum"=w520) -> ()  [unwired: 2 in, 2 out]
          n311 = property on="quit (no save)" class="Bool"("DisabledEnum"=w520) -> ()  [unwired: 2 in, 2 out]
          n312 = local write "Current Volts:"(0.0 ("Current Volts:")) -> ()
          n313 = property on="abort" class="Bool (strict)"("DisabledEnum"=2) -> ()  [unwired: 2 in, 2 out]
          n314 = local write "Bias On/Off:"(FALSE ("Visible")) -> ()
          n315 = local write "STATUS 1"("Run finished. \nSave data?" ("STATUS 1")) -> ()
        }
      }
    }
    frame #5 {
      # "*WARNING*: \"Done!\" indicator in \nFront Panel hidden."
      # "Switch off Arduino if used for T/RH measurement"
      # "Display and save data"
      n316 = global read "QC_MeasurementSetup.vi" "Rmetal Measurement Parameters"() -> (w529:T6)
      n317 = local read "Scales"() -> (w531:T1)
      n318 = local read "Iscale"() -> (w530:enum16{"Ohms", "kiloOhms", "MegaOhms"})
      n319 = while {
        shift-left: w530 -> [w562]
        shift-right: [w561] -> _
        shift-left: w531 -> [w564]
        shift-right: [w563] -> _
        tunnel: ["Quit & Save"] -> w533
        tunnel: ["quit (no save)"] -> w532
        stop <- w559 continue-if-true
        # "Loop and await decision on whether to save or junk data"
        n320 = local read "Scales"() -> (w563:T1)
        n321 = local read "Iscale"() -> (w561:enum16{"Ohms", "kiloOhms", "MegaOhms"})
        n322 = Not Equal?(x=w564, y=w563) -> (x != y?=w557:bool)
        n323 = Not Equal?(x=w562, y=w561) -> (x != y?=w556:bool)
        n324 = case shown="True" w557 {
          tunnel: w563 -> [_ w589]
          frame False {
          }
          frame True {
            # "Allow to change the IV plot representation (Linear=0, Logarithmic=1)"
            n325 = case shown="..\"Lin - Lin\"" w589 {
              tunnel: [w590 1 0 w595] -> w588
              tunnel: [w590 0 1 w595] -> w587
              frame .."Lin - Lin" {
                w590 = 0
              }
              frame "Log - Lin" {
              }
              frame "Lin - Log" {
              }
              frame "Log - log".. {
                w595 = 1
              }
            }
            n326 = property on="Igraph" class="XYGraph (strict)"("X Scale.Mapping Mode"=w588) -> ()  [unwired: 2 in, 2 out]
            n327 = property on="Igraph" class="XYGraph (strict)"("Y Scale.Mapping Mode"=w587, "YScale.Minimum"=w587) -> ()  [unwired: 2 in, 2 out]
          }
        }
        n328 = case shown="True" w556 {
          tunnel: w561 -> [_ w575]
          frame False {
          }
          frame True {
            w568 = T3."Read Array" ("Action")
            # "Set minimum in Current (Y) axis in 0 if linear and 1 if logarithmic"
            # "Allow to change the Current scale (nA, µA or mA)"
            n329 = global read "QC_MeasurementSetup.vi" "Rmetal Measurement Parameters"() -> (w570:T6)
            n330 = property on="Igraph" class="XYGraph (strict)"() -> ("YScale.Mapping Mode"=w571:u8)  [unwired: 2 in, 2 out]
            n331 = property on="Igraph" class="XYGraph (strict)"("YScale.Minimum"=w571) -> ()  [unwired: 2 in, 2 out]
            n332 = Unbundle By Name(w570) -> ("Number Of Steps"=w565:u32)
            n333 = call "IVData.vi"("Action"=w568, "Array No."=u32 1 ("Action")) -> ("Array OUT"=w577:dbl[])  [unwired: 3 in, 1 out]
            n334 = Array Subset(array=w577, index=0, length=w565) -> (w574:dbl[])
            n335 = Absolute Value(x=w574) -> (abs(x)=w573:dbl[])
            n336 = call "IVData.vi"("Action"=w568, "Array No."=u32 0 ("Action")) -> ("Array OUT"=w567:dbl[])  [unwired: 3 in, 1 out]
            n337 = case shown="..\"Ohms\"" w575 {
              tunnel: [w580 w581 w585] -> w579
              tunnel: w573 -> [w580 w583 w586]
              frame .."Ohms" {
              }
              frame "kiloOhms" {
                n338 = Divide(x=w583, y=1000.0) -> (x/y=w581:dbl[])
              }
              frame "MegaOhms".. {
                n339 = Divide(x=w586, y=1000000.0) -> (x/y=w585:dbl[])
              }
            }
            n340 = Absolute Value(x=w567) -> (abs(x)=w566:dbl[])
            n341 = Bundle(w566, w579) -> (w576:cluster{dbl[], dbl[]})  [unwired: 1 in]
            n342 = local write "Igraph"(w576) -> ()
          }
        }
        n343 = Not Or(1:"quit (no save)", 2:"Quit & Save") -> (0:w559:bool)
      }
      n344 = Unbundle By Name(w529) -> ("Temperature Readout"=w528:enum16{"Read Arduino", "Enter manually"}, "Arduino"=w522:refnum<class "ArduinoControl.lvclass">)
      n345 = case shown="\"Read Arduino\"" w528 {
        tunnel: w522 -> [_ w555]
        frame "Enter manually", Default {
        }
        frame "Read Arduino" {
          n346 = call "ArduinoClose.vi"("ArduinoControl in"=w555) -> ()  [unwired: 9 in, 2 out]
        }
      }
      n347 = case shown="True" w532 {
        tunnel: [FALSE w597] -> w534
        frame False {
        }
        frame True {
          n348 = Two Button Dialog(message="Are you sure you don't want to save the data?", 1:"Quit" ("F button name (\"Cancel\")"), 2:"Save data" ("T button name (\"OK\")")) -> (T button?=w597:bool)
        }
      }
      n349 = Or(x=w533, y=w534) -> (x .or. y?=w527:bool)
      n350 = flat-sequence {
        tunnel: w527 -> [w535]
        tunnel: [w535] -> w523
        tunnel: [TRUE] -> w521
        frame #0 {
          n351 = case shown="True" w535 {
            frame False {
            }
            frame True {
              w539 = T3."Read Array" ("Action")
              # "Show \"Saving Data ...\" message"
              # "Save data in file"
              n352 = local write "STATUS 1"("Saving Data ...") -> ()
              n353 = call "IVData.vi"("Action"=w539, "Array No."=u32 0 ("Action")) -> ("Array OUT"=w547:dbl[])  [unwired: 3 in, 1 out]
              n354 = call "IVData.vi"("Action"=w539, "Array No."=u32 5 ("Action")) -> ("Array OUT"=w538:dbl[])  [unwired: 3 in, 1 out]
              n355 = call "IVData.vi"("Action"=w539, "Array No."=u32 1 ("Action")) -> ("Array OUT"=w546:dbl[])  [unwired: 3 in, 1 out]
              n356 = Build Array(w547, w546, w538) -> (w545:dbl[][])
              n357 = Transpose 2D Array(2D array=w545) -> (transposed array=w544:dbl[][])
              n358 = call "IVData.vi"("Action"=w539, "Array No."=u32 2 ("Action")) -> ("Array OUT"=w553:dbl[])  [unwired: 3 in, 1 out]
              n359 = call "IVData.vi"("Action"=w539, "Array No."=u32 3 ("Action")) -> ("Array OUT"=w552:dbl[])  [unwired: 3 in, 1 out]
              n360 = call <vilib>:"Std Deviation and Variance.vi"("X"=w553) -> ("mean"=w542:dbl)  [unwired: 1 in, 2 out]
              n361 = call <vilib>:"Std Deviation and Variance.vi"("X"=w552) -> ("mean"=w543:dbl)  [unwired: 1 in, 2 out]
              n362 = call "SaveDataFile.vi"("Data Array"=w544, "Temperature"=w543, "Humidity"=w542, "Array Titles"="Current[uA] Resistance[Ohms]Voltage[nA]", "Strip Segment"="") -> ()  [unwired: 7 in, 4 out]
            }
          }
        }
      }
      n363 = Select(t="Run finished.\nData saved." ("STATUS 1"), s=w523, f="Run finished.\nData not saved." ("STATUS 1")) -> (s? t:f=w526:string)
      n364 = local write "STATUS 1"(w526) -> ()
      "Done!" <- w521
    }
  }
